vi "SendtoSlack.vi"(8 "error in (no error)":errorcluster, 9 "buffer":string="Test", 10 "url":string="https://hooks.slack.com/services/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") -> (0 "error out":errorcluster, 1 "body":string, 2 "headers":string)   [LabVIEW 2013]
uses:
  <vilib>/httpClient/POSTBuffer.vi
  <vilib>/httpClient/LabVIEWHTTPClient.lvlib
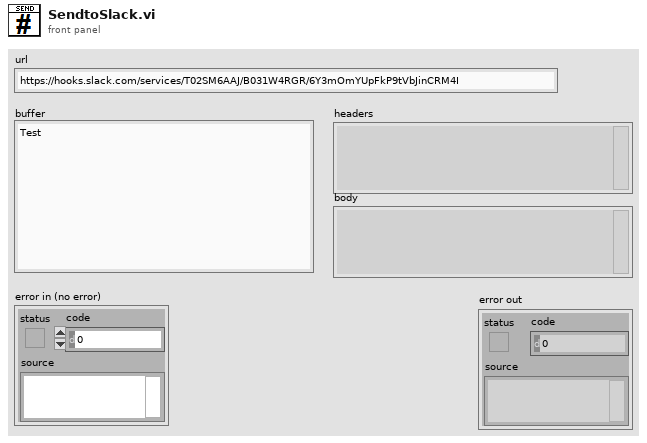
[diagram p1: front panel]
types:
  T1 = typedef "LabVIEWHTTPClient.lvlib/ClientHandle.ctl" = refnum<k1>
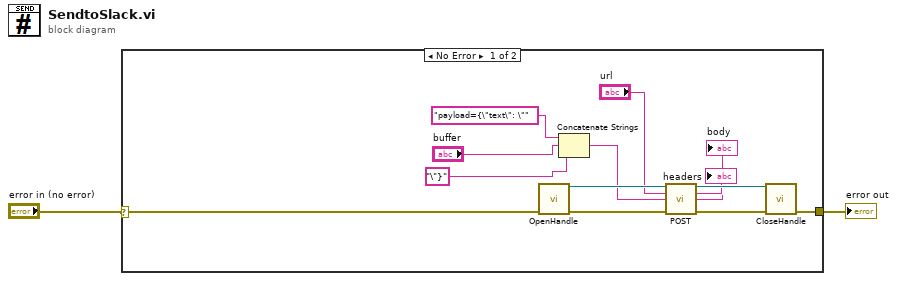
[diagram p0: block diagram]
diagram:
  n1 = case shown="No Error" "error in (no error)" {
    selector: "error in (no error)" -> [w4 w16]
    tunnel: [w9 w16] -> w2
    frame No Error {
      n2 = call <vilib>:"OpenHandle.vi"("error in (no error)"=w4) -> ("client handle out"=w15:T1, "error out"=w12:errorcluster)  [unwired: 13 in]
      n3 = Concatenate Strings("payload={\"text\": \"" ("buffer"), "buffer", "\"}" ("buffer")) -> (w5:string)
      n4 = call-poly <vilib>:"POST.vi"("client handle"=w15, "url"="url", "buffer"=w5, "error in (no error)"=w12) -> ("client handle out"=w14:T1, "headers"=→"headers":string, "body"=→"body":string, "error out"=w13:errorcluster)  [unwired: 8 in]
      n5 = call <vilib>:"CloseHandle.vi"("client handle"=w14, "error in (no error)"=w13) -> ("error out"=w9:errorcluster)  [unwired: 13 in]
    }
    frame Error {
    }
  }
  "error out" <- w2
